vi "Create Config JSON.vi"() -> ()   [LabVIEW 2023]
uses:
  Plugin/ThermotronDriver/Configuration Params.ctl
  <vilib>/ADAS Replay HIL/Template Node/Plugin/Template Node/Common Configuration Params.ctl
  <vilib>/ADAS Replay HIL/AdasCommonUtilities/AdasCommonUtilities.lvlib
  8f15ed5a-ad49-4887-bb27-9da39d6e7646.vi
  <vilib>/ADAS Replay HIL/Template Node/Plugin/Template Node/Template Node.lvclass
  Plugin/ThermotronDriver/ThermotronDriver.lvclass
panel:
  out "Version":string
  out "Generated JSON string":string
  out "error out":errorcluster
  in  "Custom Parameters":T1={"Common"={"Iteration Interval (s)"=0.001, "T0 (ns)"=0, "Priority"=100, "Processor"=-2, "Wait in Ready State"=TRUE}} {"Common"."Iteration Interval (s)" format="%#_13g"}
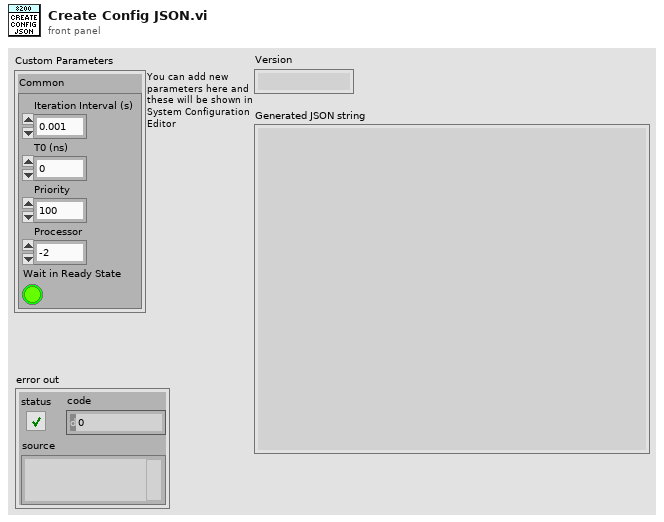
[diagram p1: front panel]
types:
  T1 = typedef "ThermotronDriver.lvlib/ThermotronDriver.lvclass/Configuration Params.ctl" = cluster{"Common":T2}
  T2 = typedef "Template Node.lvlib/Template Node.lvclass/Common Configuration Params.ctl" = cluster{"Iteration Interval (s)":dbl, "T0 (ns)":u64, "Priority":i32, "Processor":i32, "Wait in Ready State":bool}
  T3 = typedef "NI_App_Builder_API.lvlib/Build Specification Version.ctl" = cluster{"Major":u16, "Minor":u16, "Fix":u16, "Build":u16}
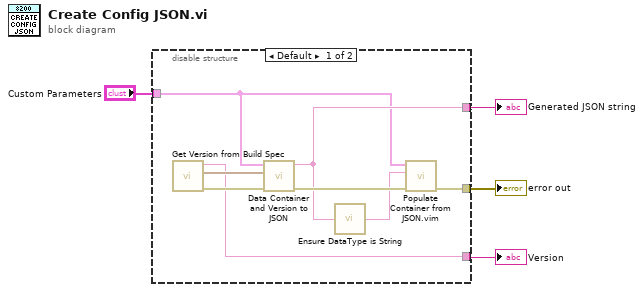
[diagram p0: block diagram]
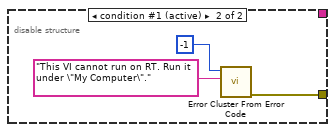
[diagram p2: hidden frame]
diagram:
  n1 = disable-structure shown="Default" {
    disable-tunnel: [w11 _] -> w4
    disable-tunnel: "Custom Parameters" -> [w10 _]
    disable-tunnel: [w9 w15] -> w2
    disable-tunnel: [w5 _] -> w1
    frame condition #0 {
      n2 = call "Get Version from Build Spec.vi"() -> ("error out"=w7:errorcluster, "Version"=w6:T3, "Version String"=w5:string)  [unwired: 8 in, 1 out]
      n3 = call <vilib>:"Data Container and Version to JSON.vi"("error in (no error)"=w7, "Version"=w6, "Container Variant"=w10) -> ("error out"=w12:errorcluster, "JSON string"=w11:string)  [unwired: 7 in]
      n4 = call <vilib>:"Ensure DataType is String.vi"("JSON In"=w11) -> ("JSON out"=w8:string)
      n5 = call "Populate Container from JSON.vim"("error in (no error)"=w12, "JSON string In"=w8, "Container In"=w10) -> ("error out"=w9:errorcluster)  [unwired: 6 in, 2 out]
    }
    frame condition #1 (active) {
      n6 = call <vilib>:"Error Cluster From Error Code.vi"("error message (\"\")"="This VI cannot run on RT. Run it under \"My Computer\"." ("error message (\"\")"), "error code (0)"=-1) -> ("error out"=w15:errorcluster)  [unwired: 7 in]
    }
  }
  "Generated JSON string" <- w4
  "error out" <- w2
  "Version" <- w1
